vi "Get content in brackets.vi"(8 "Enum":T1(ring), 10 "start":i32, 11 "String in":string) -> (2 "index out":i32=34, 3 "String out":string)   [LabVIEW 2017]
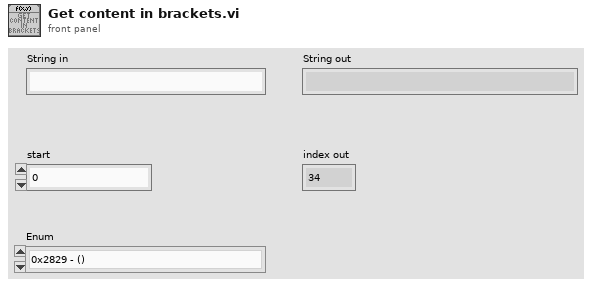
[diagram p1: front panel]
types:
  T1 = enum16{"0x2829 - ()", "0x5B5D - []", "0x7B7D - {}"}
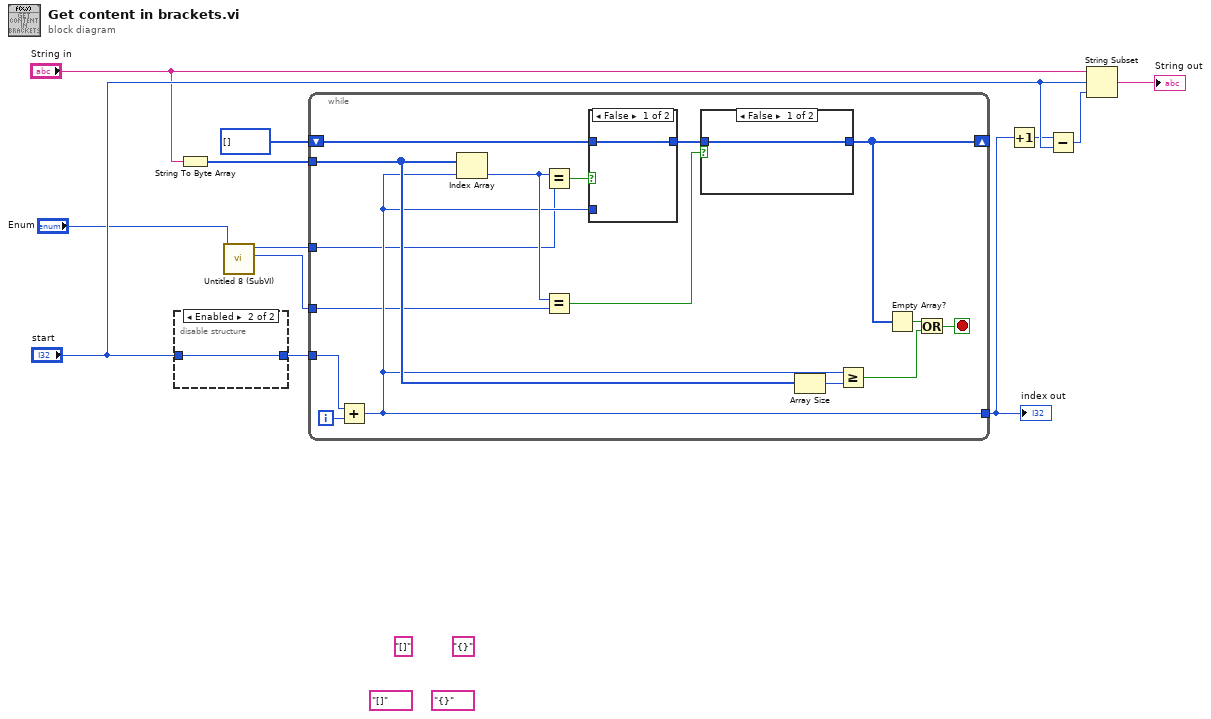
[diagram p0: block diagram]
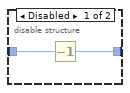
[diagram p2: hidden frame]
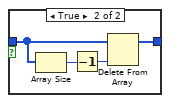
[diagram p3: hidden frame]
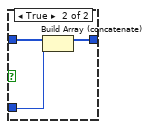
[diagram p4: hidden frame]
diagram:
  (unwired) "{}" ("String in 2")
  (unwired) "[]" ("String in 2")
  (unwired) "{}" ("String in 2")
  (unwired) "[]" ("String in 2")
  n1 = disable-structure shown="Enabled" {
    disable-tunnel: "start" -> [w14 w15]
    disable-tunnel: [w13 w15] -> w7
    frame Disabled {
      n2 = Decrement(x=w14) -> (x-1=w13:i32)
    }
    frame Enabled {
    }
  }
  n3 = String To Byte Array(string="String in") -> (unsigned byte array=w5:u8[])
  n4 = call "Untitled 8 (SubVI).vi"("Enum"="Enum") -> ("Numeric"=w1:u8, "Numeric 2"=w2:u8)  [unwired: 9 in]
  n5 = while {
    tunnel: w5 -> [w20]
    shift-right: [w27] -> _
    shift-left: i32[] [] -> [w22]
    tunnel: [w19] -> w9
    tunnel: w7 -> [w18]
    tunnel: w2 -> [w17]
    tunnel: w1 -> [w16]
    i -> [w21]
    stop <- w26 stop-if-true
    n6 = Add(x=w18, y=w21) -> (x+y=w19:i32)
    n7 = Index Array(array=w20, index=w19) -> (element=w30:u8)
    n8 = Equal?(x=w30, y=w17) -> (x = y?=w31:bool)
    n9 = Equal?(x=w30, y=w16) -> (x = y?=w23:bool)
    n10 = case shown="False" w31 {
      tunnel: w22 -> [w37 w40]
      tunnel: w19 -> [_ w39]
      tunnel: [w37 w38] -> w29
      frame False {
      }
      frame True {
        n11 = Build Array (concatenate)(w40, w39) -> (w38:i32[])
      }
    }
    n12 = case shown="False" w23 {
      tunnel: w29 -> [w32 w35]
      tunnel: [w32 w33] -> w27
      frame False {
      }
      frame True {
        n13 = Array Size(array=w35) -> (size(s)=w36:i32)
        n14 = Decrement(x=w36) -> (x-1=w34:i32)
        n15 = Delete From Array(array=w35, index=w34) -> (array with subset deleted=w33:i32[])  [unwired: 1 in, 1 out]
      }
    }
    n16 = Array Size(array=w20) -> (size(s)=w25:i32)
    n17 = Greater Or Equal?(x=w19, y=w25) -> (x >= y?=w24:bool)
    n18 = Empty Array?(array=w27) -> (empty?=w28:bool)
    n19 = Or(x=w28, y=w24) -> (x .or. y?=w26:bool)
  }
  "index out" <- w9
  n20 = Increment(x=w9) -> (x+1=w11:i32)
  n21 = Subtract(x=w11, y="start") -> (x-y=w8:i32)
  n22 = String Subset(string="String in", offset (0)="start", length (rest)=w8) -> (substring=→"String out":string)
